vi "TestVirtual3.vi"(0 "reference in":refnum<class "G#SubClass1.lvclass">, 5 "error in (no error)":errorcluster) -> (14 "reference out":refnum<class "G#SubClass1.lvclass">, 15 "MethodName":string[](array[string]), 19 "error out":errorcluster)   [LabVIEW 2017, in "G#SubClass1.lvclass"]
uses:
  G#SubClass1.lvclass
  G#BaseClass1_class/G#BaseClass1.lvclass
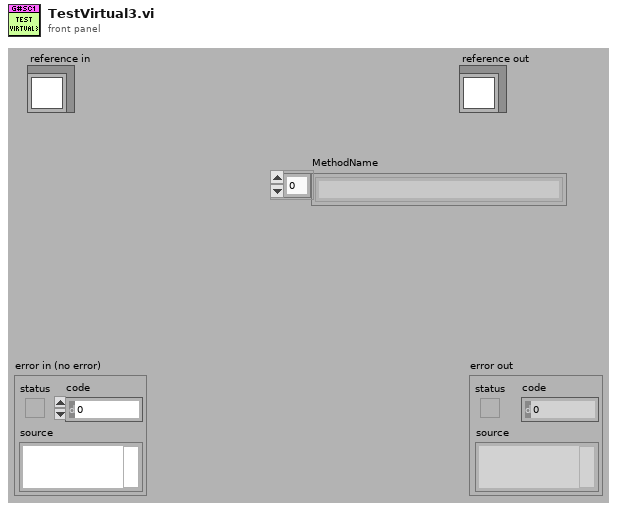
[diagram p1: front panel]
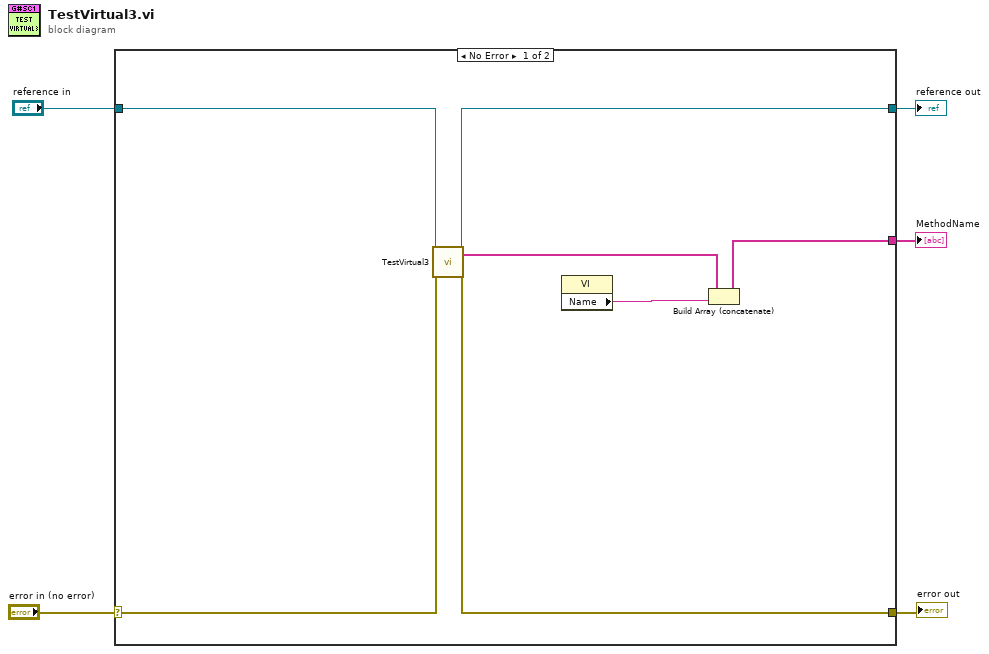
[diagram p0: block diagram]
diagram:
  n1 = case shown="No Error" "error in (no error)" {
    selector: "error in (no error)" -> [w12 w14]
    tunnel: [w11 w14] -> w4
    tunnel: [w9 w13] -> w2
    tunnel: "reference in" -> [w10 w13]
    tunnel: [w6 _] -> w1
    frame No Error {
      n2 = call-parent "TestVirtual3.vi"("reference in"=w10, "error in (no error)"=w12) -> ("reference out"=w9:refnum<class "G#SubClass1.lvclass">, "MethodName"=w7:string[], "error out"=w11:errorcluster)  [unwired: 15 in]
      n3 = property class="VI"() -> ("Name"=w8:string)  [unwired: 2 in, 2 out]
      n4 = Build Array (concatenate)(w7, w8) -> (w6:string[])
    }
    frame Error {
    }
  }
  "error out" <- w4
  "reference out" <- w2
  "MethodName" <- w1
